vi "Update Number of Analog Channels.vi"(10 "New Number":i32, 11 "UI Data in":refnum<class "Settings UI.lvclass">) -> (3 "UI Data out":refnum<class "Settings UI.lvclass">)   [LabVIEW 2024, in "Output Sequencer.lvlib" / "Settings UI.lvclass"]
uses:
  Settings UI.lvclass
  Types/Tree Index Enum.ctl
  Settings UI.lvclass/Settings UI.ctl
  Globals/Global Tree Data.vi
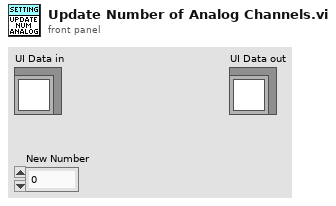
[diagram p1: front panel]
types:
  T1 = typedef "Output Sequencer.lvlib/Settings UI.lvclass/Tree Index Enum.ctl" = enum16{"General Settings", "Num Steps", "Num Analog", "Num Digital", "Show Confirmation", "Interp Priority", "Adv Timing", "Enable Conditions", "Seq Execution", "Reset Test Start", "Only When Test", "Delay After Test", "Start condition", "Re-triggering", "Stop condition", "Stop After Cycles", "Stop Values", "Default Values", "Default Analog", "Default Digital", "Steps", "Step #", "Description", "Precondition", "Duration", "Mode", "Delay Between Vals", "Analog Values", "Digital Values", "Postcondition", "On True", "On False"}
  T2 = typedef "Output Sequencer.lvlib/Settings UI.lvclass/Step Settings.ctl" = cluster{"Description":string, "Precondition":string, "Duration":dbl, "Mode":string, "Delay Between Values":dbl, "Analog Values":string[], "Digital Values":string[], "Postcondition":string, "On True":string, "On False":string}
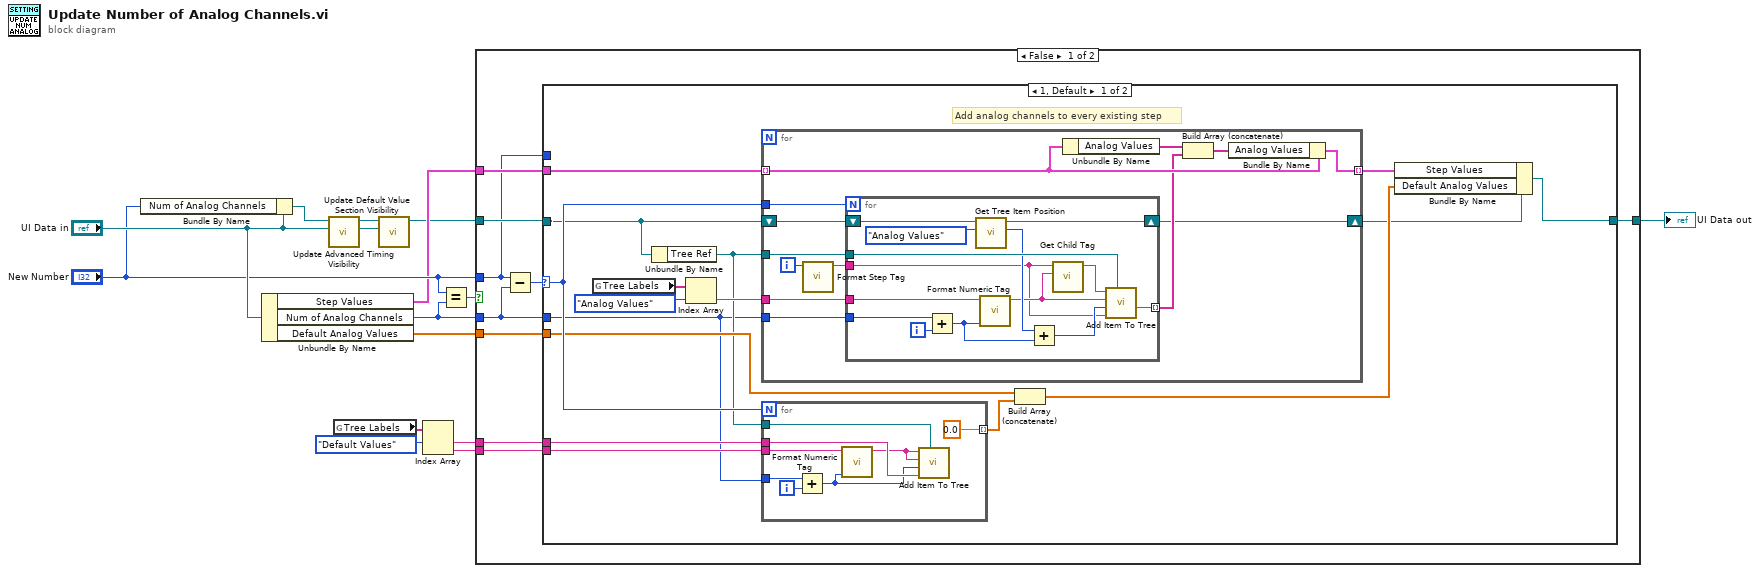
[diagram p0: block diagram]
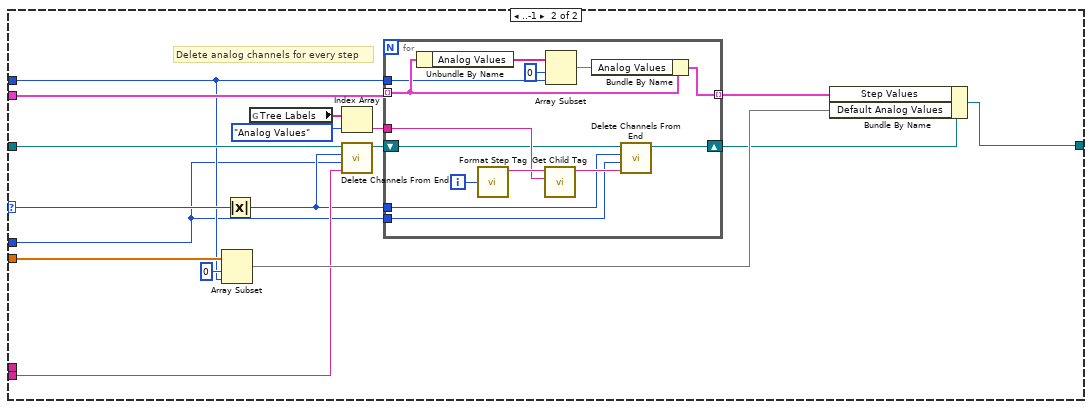
[diagram p2: hidden frame]
diagram:
  n1 = Bundle By Name(cluster="UI Data in", "Num of Analog Channels"="New Number") -> (w3:refnum<class "Settings UI.lvclass">)
  n2 = Unbundle By Name("UI Data in") -> ("Step Values"=w6:T2[], "Num of Analog Channels"=w8:i32, "Default Analog Values"=w9:dbl[])
  n3 = call "Update Advanced Timing Visibility.vi"("Previous UI Data in"="UI Data in", "New UI Data in"=w3) -> ("Previous UI Data out"=w14:refnum<class "Settings UI.lvclass">, "New UI Data out"=w2:refnum<class "Settings UI.lvclass">)  [unwired: 8 in]
  n4 = global read "Global Tree Data.vi" "Tree Labels"() -> (w10:string[])
  n5 = call "Update Default Value Section Visibility.vi"("Previous UI Data in"=w14, "New UI Data in"=w2) -> ("New UI Data out"=w1:refnum<class "Settings UI.lvclass">)  [unwired: 9 in]
  n6 = Index Array(array=w10, index #1=Tree_Index_Enum."Default Values" ("Tree Index Enum")) -> (element #1=w12:string, element #2=w11:string)  [unwired: 1 in]
  n7 = Equal?(x="New Number", y=w8) -> (x = y?=w4:bool)
  n8 = case shown="False" w4 {
    tunnel: w1 -> [w21 w107]
    tunnel: [w20 w107] -> w5
    tunnel: w8 -> [w22 _]
    tunnel: "New Number" -> [w19 _]
    tunnel: w6 -> [w23 _]
    tunnel: w9 -> [w18 _]
    tunnel: w11 -> [w17 _]
    tunnel: w12 -> [w16 _]
    frame False {
      n9 = Subtract(x=w19, y=w22) -> (x-y=w24:i32)
      n10 = case shown="1, Default" w24 {
        selector: w24 -> [w33 w91]
        tunnel: w23 -> [w40 w82]
        tunnel: w22 -> [w26 w78]
        tunnel: w21 -> [w28 w85]
        tunnel: [w36 w90] -> w20
        tunnel: w19 -> [_ w81]
        tunnel: w18 -> [w31 w89]
        tunnel: w17 -> [w34 w84]
        tunnel: w16 -> [w35 _]
        frame 1, Default {
          # "Add analog channels to every existing step"
          n11 = global read "Global Tree Data.vi" "Tree Labels"() -> (w39:string[])
          n12 = Unbundle By Name(w28) -> ("Tree Ref"=w27:refnum<vi>)
          n13 = Index Array(array=w39, index=Tree_Index_Enum."Analog Values" ("Tree Index Enum")) -> (element=w38:string)
          n14 = for {
            tunnel: w27 -> [w61]
            tunnel: w40 -> [w57] mode=indexing
            tunnel: w26 -> [w60]
            tunnel: w33 -> [w59]
            tunnel: w38 -> [w58]
            tunnel: [w53] -> w37 mode=indexing
            shift-right: [w49] -> w25
            shift-left: w28 -> [w52]
            i -> [w51]
            n15 = call "Format Step Tag.vi"("Step Number"=w51) -> ("Tag"=w50:string)  [unwired: 10 in]
            n16 = for {
              N: w59 -> [_]
              tunnel: w61 -> [w75]
              tunnel: w60 -> [w74]
              tunnel: w58 -> [w66]
              tunnel: w50 -> [w62]
              tunnel: [w71] -> w55 mode=indexing
              shift-right: [w63] -> w49
              shift-left: w52 -> [w69]
              i -> [w73]
              n17 = Add(x=w74, y=w73) -> (x+y=w65:i32)
              n18 = call "Get Tree Item Position.vi"("Step item"=Tree_Index_Enum."Analog Values", "UI Data in"=w69) -> ("Position"=w68:i32, "UI Data out"=w63:refnum<class "Settings UI.lvclass">)  [unwired: 8 in]
              n19 = call "Format Numeric Tag.vi"("Number"=w65, "Tree label"=w66) -> ("Tag"=w64:string)  [unwired: 9 in]
              n20 = Add(x=w68, y=w65) -> (x+y=w72:i32)
              n21 = call "Get Child Tag.vi"("Child label"=w64, "Parent tag"=w62) -> ("Child tag"=w67:string)  [unwired: 9 in]
              n22 = call "Add Item To Tree.vi"("TreeControl in"=w75, "Parent Tag"=w62, "Child Position"=w72, "Left Cell String"=w64, "Child Tag in"=w67) -> ("Child Text out"=w71:string)  [unwired: 6 in]
            }
            n23 = Unbundle By Name(w57) -> ("Analog Values"=w56:string[])
            n24 = Build Array (concatenate)(w56, w55) -> (w54:string[])
            n25 = Bundle By Name(cluster=w57, "Analog Values"=w54) -> (w53:T2)
          }
          n26 = for {
            N: w33 -> [_]
            tunnel: w27 -> [w48]
            tunnel: w35 -> [w45]
            tunnel: w34 -> [w42]
            tunnel: w26 -> [w46]
            tunnel: [0.0] -> w32 mode=indexing
            i -> [w47]
            n27 = Add(x=w46, y=w47) -> (x+y=w43:i32)
            n28 = call "Format Numeric Tag.vi"("Number"=w43, "Tree label"=w42) -> ("Tag"=w41:string)  [unwired: 9 in]
            n29 = call "Add Item To Tree.vi"("TreeControl in"=w48, "Parent Tag"=w45, "Child Position"=w43, "Left Cell String"=w41, "Child Tag in"=w41) -> ()  [unwired: 6 in, 1 out]
          }
          n30 = Build Array (concatenate)(w31, w32) -> (w30:dbl[])
          n31 = Bundle By Name(cluster=w25, "Step Values"=w37, "Default Analog Values"=w30) -> (w36:refnum<class "Settings UI.lvclass">)
        }
        frame ..-1 {
          # "Delete analog channels for every step"
          n32 = Array Subset(array=w89, index=0, length=w81) -> (w87:dbl[])
          n33 = Absolute Value(x=w91) -> (abs(x)=w79:i32)
          n34 = global read "Global Tree Data.vi" "Tree Labels"() -> (w92:string[])
          n35 = Index Array(array=w92, index=Tree_Index_Enum."Analog Values" ("Tree Index Enum")) -> (element=w80:string)
          n36 = call "Delete Channels From End.vi"("Channel Label"=w84, "Prior Number of Channels"=w78, "Number of Channels to Delete"=w79, "UI Data in"=w85) -> ("UI Data out"=w83:refnum<class "Settings UI.lvclass">)  [unwired: 7 in]
          n37 = for {
            tunnel: w82 -> [w106] mode=indexing
            tunnel: w78 -> [w95]
            tunnel: w79 -> [w94]
            tunnel: w80 -> [w98]
            tunnel: [w105] -> w76 mode=indexing
            tunnel: w81 -> [w102]
            shift-right: [w93] -> w77
            shift-left: w83 -> [w97]
            i -> [w100]
            n38 = Unbundle By Name(w106) -> ("Analog Values"=w104:string[])
            n39 = call "Format Step Tag.vi"("Step Number"=w100) -> ("Tag"=w99:string)  [unwired: 10 in]
            n40 = call "Get Child Tag.vi"("Child label"=w98, "Parent tag"=w99) -> ("Child tag"=w96:string)  [unwired: 9 in]
            n41 = Array Subset(array=w104, index=0, length=w102) -> (w103:string[])
            n42 = Bundle By Name(cluster=w106, "Analog Values"=w103) -> (w105:T2)
            n43 = call "Delete Channels From End.vi"("Channel Label"=w96, "Prior Number of Channels"=w95, "Number of Channels to Delete"=w94, "UI Data in"=w97) -> ("UI Data out"=w93:refnum<class "Settings UI.lvclass">)  [unwired: 7 in]
          }
          n44 = Bundle By Name(cluster=w77, "Step Values"=w76, "Default Analog Values"=w87) -> (w90:refnum<class "Settings UI.lvclass">)
        }
      }
    }
    frame True {
    }
  }
  "UI Data out" <- w5
